vi "KM_Lockin.vi"() -> ()   [LabVIEW 2015]
uses:
  Dropbox/MaxPlanck/HF2LI_KM/MQM Data Transfer_KM.vi
  <vilib>/Utility/file.llb/Write To Spreadsheet File (string).vi
  <vilib>/Utility/file.llb/Write To Spreadsheet File (DBL).vi
  Dropbox/MaxPlanck/HF2LI_KM/String Array Select.vi
  Dropbox/MaxPlanck/HF2LI_KM/Numeric Array Select.vi
panel:
  in  "Tab Control":enum32{"Display Data", "Sweep Arming"}(tab)
  in  "Control":bool=TRUE
  in  "Stop":bool=TRUE
  out "XY Graph":cluster{dbl[], dbl[]}[](graph)
  in  "Display Elements":cluster{"X":bool, "Y":bool, "Name":u16}[](array[cluster]) {"Name" items=["Time (ms)", "Field (T)", "Temperature (K)", "", "HFLI_1.0 Freq (Hz)", "HFLI_1.0 R (V)", "HFLI_1.0 Theta (deg)", "HFLI_1.0 X (mV)", "HFLI_1.0 Y (mV)"]}
  in  "X-Axis":u16(ring) items=["Linear", "Reciprocal", "Log10"]
  in  "Filename":path=path "C:/Users/putkonen.CPFS/Dropbox.lvm"
  in  "Delay (ms)":dbl=2000.0
  out "Data Rate (ms)":u32
  in  "Finish":bool
  in  "Y-Axis":u16(ring) items=["Linear", "Reciprocal", "Log10"]
  in  "Data Recording":bool=TRUE
  in  "DAQ time (ms)":u32=500
  out "Circles":cluster{dbl[], dbl[]}(graph)
  in  "X":u16(ring) items=["Linear", "Reciprocal", "Log10"]
  in  "Y":u16(ring) items=["Linear", "Reciprocal", "Log10"]
  out "Phase":cluster{dbl[], dbl[]}(graph)
  in  "Frequency":u16(ring) items=["Linear", "Reciprocal", "Log10"]
  in  "Theta":u16(ring) items=["Linear", "Reciprocal", "Log10"]
  out "# pts in freq sweep":i32
  out "Data Rate  (ms)":u32
  in  "DAQ time (ms)":u32=50
  in  "Fequency sweep datafile":path=path "C:/Users/putkonen.CPFS/Dropbox.lvm" caption="Filename"
  in  "Start (Hz)":dbl=48.29
  in  "Stop (Hz)":dbl=48.57
  in  "# pts in scan":dbl=100.0
  in  "Bandwidth (Hz)":dbl=10.0
  out "Global Stop":bool
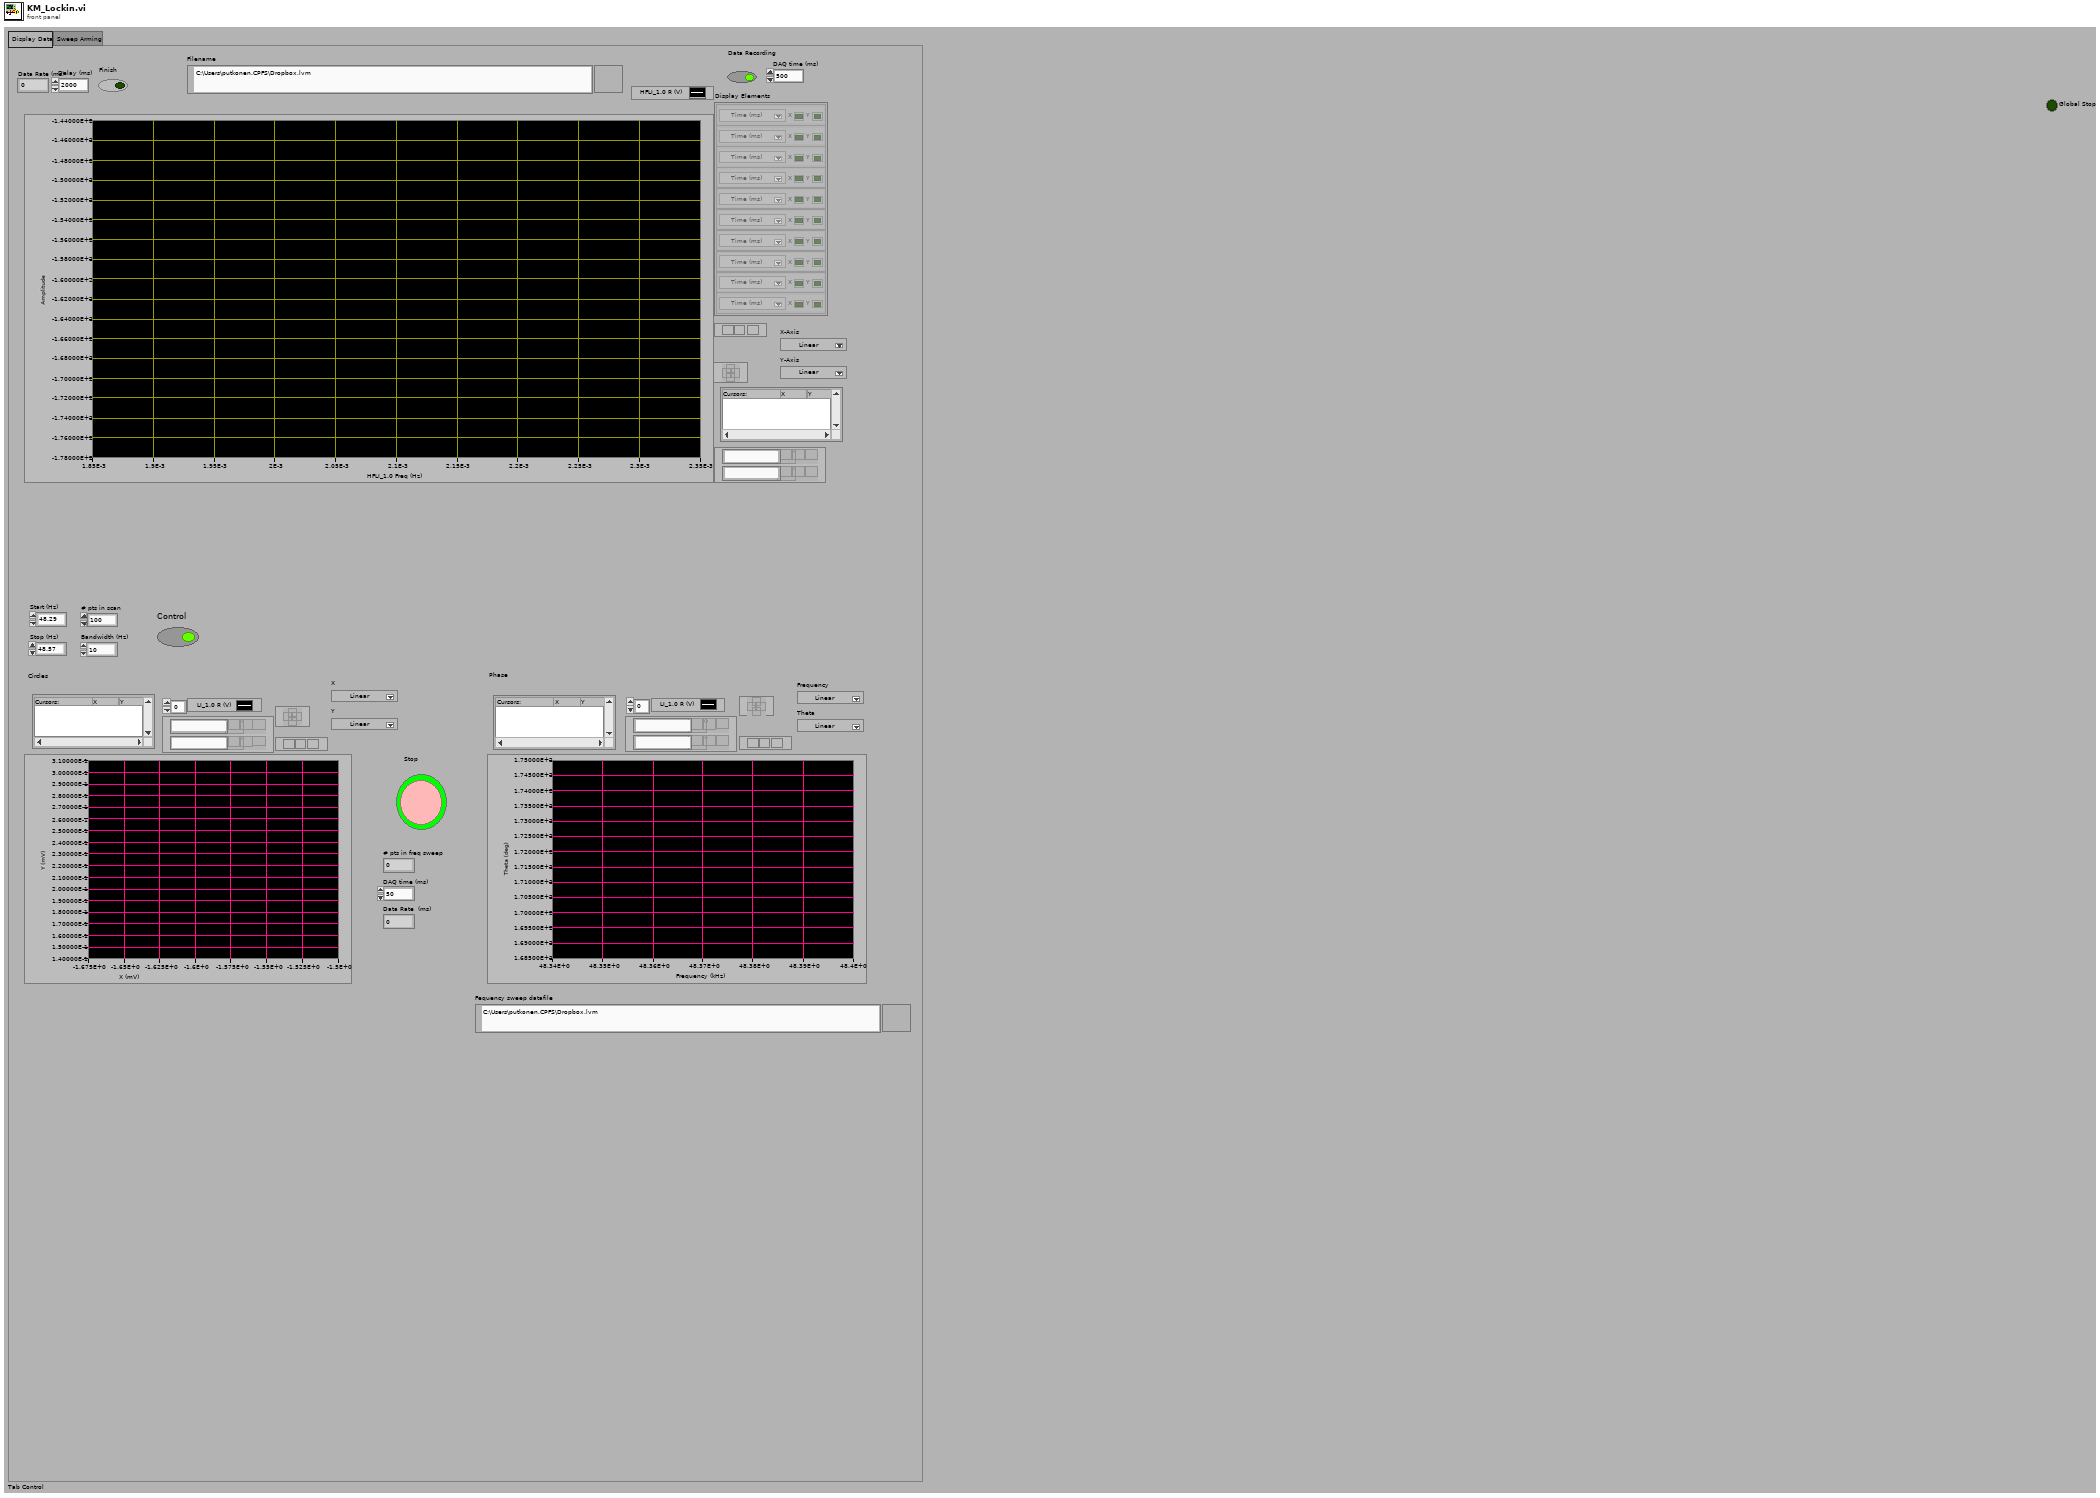
[diagram p1: front panel]
types:
  T1 = typedef "ZI_Frontpanel.ctl" = cluster{"Lockin 1 Demod 0":cluster{"R(V)":dbl, "Theta (deg)":dbl, "Timestamp (ms)":u32}, "Lockin 2 Demod 0":cluster{"R(V)":dbl, "Theta (deg)":dbl, "Timestamp (ms)":u32}, "Lockin 3 Demod 0":cluster{"R(V)":dbl, "Theta (deg)":dbl, "Timestamp (ms)":u32}, "Lockin 4 Demod 0":cluster{"R(V)":dbl, "Theta (deg)":dbl, "Timestamp (ms)":u32}, "Lockin 1 Demod 1":cluster{"R(V)":dbl, "Theta (deg)":dbl, "Timestamp (ms)":u32}, "Lockin 2 Demod 1":cluster{"R(V)":dbl, "Theta (deg)":dbl, "Timestamp (ms)":u32}, "Lockin 3 Demod 1":cluster{"R(V)":dbl, "Theta (deg)":dbl, "Timestamp (ms)":u32}, "Lockin 4 Demod 1":cluster{"R(V)":dbl, "Theta (deg)":dbl, "Timestamp (ms)":u32}, "Lockin 1 Demod 2":cluster{"R(V)":dbl, "Theta (deg)":dbl, "Timestamp (ms)":u32}, "Lockin 1 Demod 3":cluster{"R(V)":dbl, "Theta (deg)":dbl, "Timestamp (ms)":u32}, "LI1 active":bool, "LI2 active":bool, "LI3 active":bool, "LI4 active":bool}
  T2 = typedef "HF_FrontPanel.ctl" = cluster{"Lockin 1 Demod 0":cluster{"R(V)":dbl, "Theta (deg)":dbl, "Frequency (Hz)":dbl, "X (mV)":dbl, "Y (mV)":dbl}, "LI1 active":bool, "Timestamp (ms)":u32}
  T3 = typedef "PPMS_Status.ctl" = cluster{"Field":cluster{"Field (T)":dbl, "Field stable":bool, "Timestamp (ms)":u32}, "Temperature":cluster{"Temperature (K)":dbl, "Temperature stable":bool, "Timestamp (ms)":u32}}
  T4 = cluster{"Request new file":bool, "Sweep variable":u16, "Pause DAQ":bool}
  T5 = typedef "Rotator_Status.ctl" = cluster{"Angle (deg)":dbl, "Stopped":bool, "Timestamp (ms)":u32}
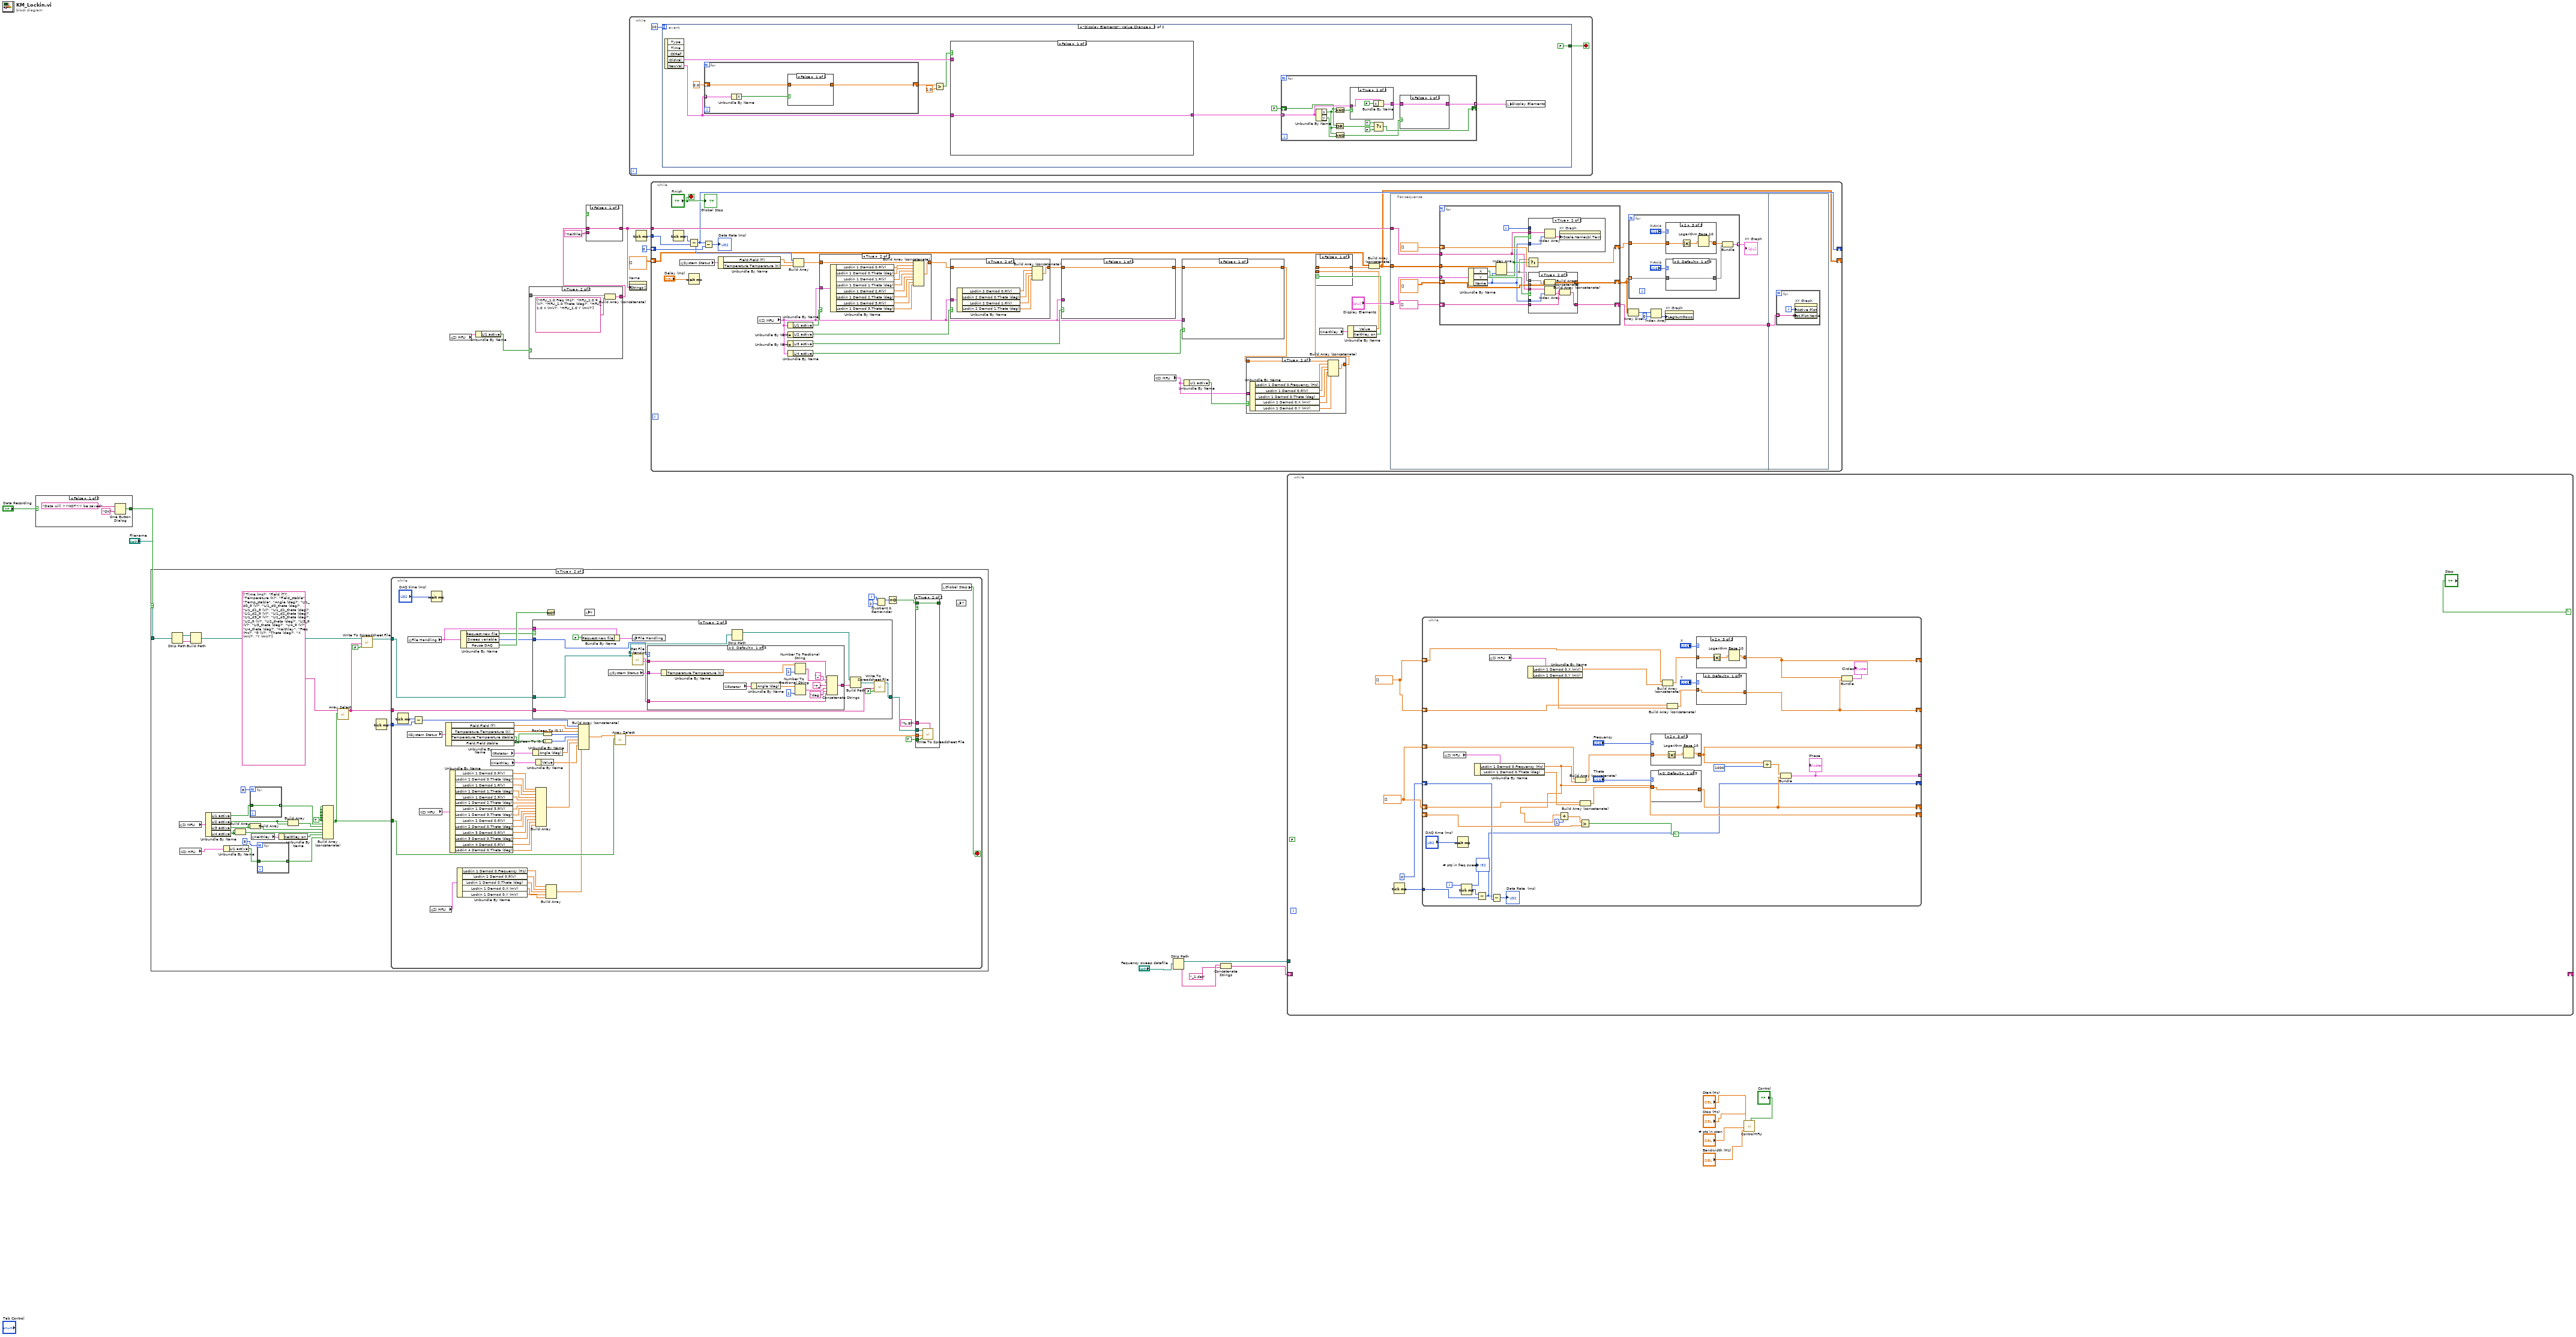
[diagram p0: block diagram]
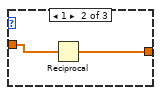
[diagram p2: hidden frame]
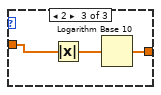
[diagram p3: hidden frame]
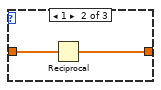
[diagram p5: hidden frame]
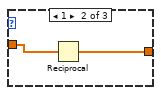
[diagram p6: hidden frame]
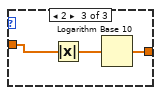
[diagram p7: hidden frame]
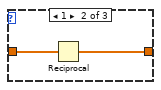
[diagram p9: hidden frame]
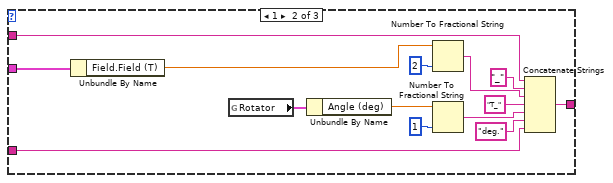
[diagram p13: hidden frame]
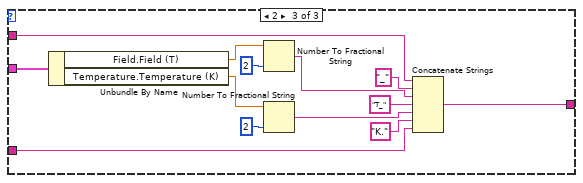
[diagram p14: hidden frame]
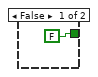
[diagram p15: hidden frame]
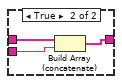
[diagram p17: hidden frame]
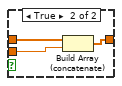
[diagram p19: hidden frame]
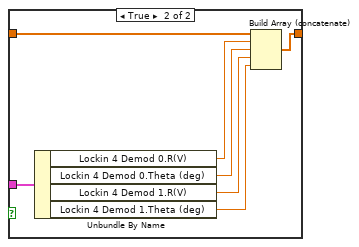
[diagram p20: hidden frame]
diagram:
  n1 = case shown="False" "Data Recording" {
    selector: "Data Recording" -> [_ w26]
    tunnel: [w23 w26] -> w15
    frame False {
      n2 = One Button Dialog(message="Data will >>NOT<< be saved", button name ("OK")="OK") -> (true=w23:bool)
    }
    frame True {
    }
  }
  n3 = case shown="True" w15 {
    tunnel: "Filename" -> [_ w53]
    frame False {
    }
    frame True {
      w45 = TRUE
      n4 = Strip Path(path=w53) -> (stripped path=w49:path, name=w47:string)
      n5 = global read "MQM Data Transfer_KM.vi" "ZI MFLI"() -> (w44:T1)
      n6 = global read "MQM Data Transfer_KM.vi" "ZI HFLI"() -> (w30:T2)
      n7 = Build Path(base path=w49, name or relative path=w47) -> (appended path=w50:path)
      n8 = Unbundle By Name(w44) -> ("LI1 active"=w43:bool, "LI2 active"=w40:bool, "LI3 active"=w39:bool, "LI4 active"=w38:bool)
      n9 = Unbundle By Name(w30) -> ("LI1 active"=w29:bool)
      n10 = Build Array(w38, w38) -> (w35:bool[])
      n11 = for {
        N: 8 -> [_]
        tunnel: w43 -> [w55]
        tunnel: [w55] -> w41 mode=indexing
      }
      n12 = Build Array(w39, w39) -> (w36:bool[])
      n13 = global read "MQM Data Transfer_KM.vi" "Keithley"() -> (w34:cluster{"Value":dbl, "Keithley on":bool})
      n14 = for {
        N: 5 -> [_]
        tunnel: w29 -> [w54]
        tunnel: [w54] -> w27 mode=indexing
      }
      n15 = Unbundle By Name(w34) -> ("Keithley on"=w33:bool)
      n16 = Build Array(w40, w40) -> (w37:bool[])
      n17 = Build Array (concatenate)(w45, w45, w45, w45, w45, w45, w41, w37, w36, w35, w33, w27) -> (w32:bool[])
      n18 = call-poly "Array Select.vi"("Selector array"=w32, "Full array"=string[] ["Time (ms)", "Field (T)", "Temperature (K)", "Field_stable", "Temp_stable", "Angle (deg)", "LI1_d0_R (V)", "LI1_d0_theta (deg)", "LI1_d1_R (V)", "LI1_d1_theta (deg)", "LI1_d2_R (V)", "LI1_d2_theta (deg)", "LI1_d3_R (V)", "LI1_d3_theta (deg)", "LI2_R (V)", "LI2_theta (deg)", "LI3_R (V)", "LI3_theta (deg)", "LI4_R (V)", "LI4_theta (deg)", "Keithley", "Freq (Hz)", "R (V)", "Theta (deg)", "X (mV)", "Y (mV)"]) -> ("Array"=w31:string[])  [unwired: 9 in]
      n19 = call-poly <vilib>:"Write To Spreadsheet File.vi"("append to file? (new file:F)"=FALSE, "1D data"=w31, "file path (dialog if empty)"=w50) -> ("new file path (Not A Path if cancelled)"=w48:path)  [unwired: 5 in]
      n20 = Tick Count (ms)() -> (millisecond timer value=w52:u32)
      n21 = while {
        tunnel: w52 -> [w110]
        tunnel: w48 -> [w70]
        tunnel: w32 -> [w77]
        tunnel: w31 -> [w67]
        i -> [w76]
        stop <- w102 stop-if-true
        n22 = Tick Count (ms)() -> (millisecond timer value=w108:u32)
        n23 = global read "MQM Data Transfer_KM.vi" "System Status"() -> (w109:T3)
        n24 = global read "MQM Data Transfer_KM.vi" "File Handling"() -> (w66:T4)
        n25 = Subtract(x=w108, y=w110) -> (x-y=w107:u32)
        n26 = global read "MQM Data Transfer_KM.vi" "ZI MFLI"() -> (w98:T1)
        n27 = global read "MQM Data Transfer_KM.vi" "ZI HFLI"() -> (w63:T2)
        n28 = Wait (ms)(milliseconds to wait="DAQ time (ms)") -> ()  [unwired: 1 out]
        n29 = Unbundle By Name(w109) -> ("Field.Field (T)"=w106:dbl, "Temperature.Temperature (K)"=w105:dbl, "Temperature.Temperature stable"=w86:bool, "Field.Field stable"=w88:bool)
        n30 = Unbundle By Name(w98) -> ("Lockin 1 Demod 0.R(V)"=w97:dbl, "Lockin 1 Demod 0.Theta (deg)"=w96:dbl, "Lockin 1 Demod 1.R(V)"=w95:dbl, "Lockin 1 Demod 1.Theta (deg)"=w94:dbl, "Lockin 1 Demod 2.R(V)"=w93:dbl, "Lockin 1 Demod 2.Theta (deg)"=w92:dbl, "Lockin 1 Demod 3.R(V)"=w91:dbl, "Lockin 1 Demod 3.Theta (deg)"=w90:dbl, "Lockin 2 Demod 0.R(V)"=w89:dbl, "Lockin 2 Demod 0.Theta (deg)"=w82:dbl, "Lockin 3 Demod 0.R(V)"=w81:dbl, "Lockin 3 Demod 0.Theta (deg)"=w80:dbl, "Lockin 4 Demod 0.R(V)"=w79:dbl, "Lockin 4 Demod 0.Theta (deg)"=w78:dbl)
        n31 = Unbundle By Name(w63) -> ("Lockin 1 Demod 0.Frequency (Hz)"=w62:dbl, "Lockin 1 Demod 0.R(V)"=w61:dbl, "Lockin 1 Demod 0.Theta (deg)"=w60:dbl, "Lockin 1 Demod 0.X (mV)"=w59:dbl, "Lockin 1 Demod 0.Y (mV)"=w58:dbl)
        n32 = Unbundle By Name(w66) -> ("Request new file"=w71:bool, "Sweep variable"=w68:u16, "Pause DAQ"=w73:bool)
        n33 = global read "MQM Data Transfer_KM.vi" "Keithley"() -> (w99:cluster{"Value":dbl, "Keithley on":bool})
        n34 = global read "MQM Data Transfer_KM.vi" "Rotator"() -> (w100:T5)
        n35 = case shown="True" w71 {
          tunnel: w70 -> [w111 w122]
          tunnel: [w111 w115] -> w69
          tunnel: w68 -> [_ w124]
          tunnel: w67 -> [_ w117]
          tunnel: w66 -> [_ w114]
          frame False {
          }
          frame True {
            n36 = Bundle By Name(cluster=w114, "Request new file"=FALSE) -> (w112:T4)
            n37 = global read "MQM Data Transfer_KM.vi" "System Status"() -> (w123:T3)
            n38 = global write "MQM Data Transfer_KM.vi" "File Handling"(w112) -> ()
            n39 = call <vilib>:"Get File Extension.vi"("file"=w122) -> ("filename without extension"=w121:string, "lowercase file extension"=w120:string)  [unwired: 6 in, 3 out]
            n40 = case shown="0, Default" w124 {
              tunnel: w123 -> [w139 w148 w159]
              tunnel: w121 -> [w136 w149 w161]
              tunnel: w120 -> [w126 w140 w154]
              tunnel: [w132 w146 w160] -> w119
              frame 0, Default {
                n41 = Unbundle By Name(w139) -> ("Temperature.Temperature (K)"=w138:dbl)
                n42 = global read "MQM Data Transfer_KM.vi" "Rotator"() -> (w131:T5)
                n43 = Unbundle By Name(w131) -> ("Angle (deg)"=w129:dbl)
                n44 = Number To Fractional String(number=w138, precision (6)=i16 2) -> (F-format string=w134:string)  [unwired: 2 in]
                n45 = Number To Fractional String(number=w129, precision (6)=i16 1) -> (F-format string=w128:string)  [unwired: 2 in]
                n46 = Concatenate Strings(w136, "_", w134, "T_", w128, "deg." ("string"), w126) -> (w132:string)
              }
              frame 1 {
                n47 = Unbundle By Name(w148) -> ("Field.Field (T)"=w147:dbl)
                n48 = global read "MQM Data Transfer_KM.vi" "Rotator"() -> (w145:T5)
                n49 = Unbundle By Name(w145) -> ("Angle (deg)"=w143:dbl)
                n50 = Number To Fractional String(number=w147, precision (6)=i16 2) -> (F-format string=w151:string)  [unwired: 2 in]
                n51 = Number To Fractional String(number=w143, precision (6)=i16 1) -> (F-format string=w142:string)  [unwired: 2 in]
                n52 = Concatenate Strings(w149, "_", w151, "T_", w142, "deg." ("string"), w140) -> (w146:string)
              }
              frame 2 {
                n53 = Unbundle By Name(w159) -> ("Field.Field (T)"=w166:dbl, "Temperature.Temperature (K)"=w157:dbl)
                n54 = Number To Fractional String(number=w166, precision (6)=i16 2) -> (F-format string=w163:string)  [unwired: 2 in]
                n55 = Number To Fractional String(number=w157, precision (6)=i16 2) -> (F-format string=w156:string)  [unwired: 2 in]
                n56 = Concatenate Strings(w161, "_", w163, "T_", w156, "K." ("string"), w154) -> (w160:string)
              }
            }
            n57 = Strip Path(path=w122) -> (stripped path=w125:path)  [unwired: 1 out]
            n58 = Build Path(base path=w125, name or relative path=w119) -> (appended path=w116:path)
            n59 = call-poly <vilib>:"Write To Spreadsheet File.vi"("append to file? (new file:F)"=FALSE, "1D data"=w117, "file path (dialog if empty)"=w116) -> ("new file path (Not A Path if cancelled)"=w115:path)  [unwired: 5 in]
          }
        }
        n60 = Unbundle By Name(w100) -> ("Angle (deg)"=w84:dbl)
        n61 = Build Array(w97, w96, w95, w94, w93, w92, w91, w90, w89, w82, w81, w80, w79, w78) -> (w83:dbl[])
        n62 = Unbundle By Name(w99) -> ("Value"=w64:dbl)
        n63 = Boolean To (0,1)(Boolean=w88) -> (0, 1=w87:i16)
        n64 = Boolean To (0,1)(Boolean=w86) -> (0, 1=w85:i16)
        n65 = Not(x=w73) -> ()  [unwired: 1 out]
        n66 = Build Array(w62, w61, w60, w59, w58) -> (w57:dbl[])
        n67 = Build Array (concatenate)(w107, w106, w105, w87, w85, w84, w83, w64, w57) -> (w65:dbl[])
        n68 = local read item#-1() -> ()  [unwired: 1 in]
        n69 = call-poly "Array Select.vi"("Selector array"=w77, "Full array"=w65) -> ("Array"=w56:dbl[])  [unwired: 9 in]
        n70 = Quotient & Remainder(x=w76, y=2) -> (x-y*floor(x/y)=w74:i32)  [unwired: 1 out]
        n71 = Equal To 0?(x=w74) -> (x = 0?=w72:bool)
        n72 = case shown="True" {
          selector: _ -> [_ _]
          tunnel: TRUE ("append to file? (new file:F)") -> [_ w172]
          tunnel: "%.8f" ("format (%.3f)") -> [_ w171]
          tunnel: w56 -> [_ w170]
          tunnel: w72 -> [_ w169]
          tunnel: [FALSE w169] -> _
          tunnel: w69 -> [_ w168]
          frame False {
          }
          frame True {
            n73 = call-poly <vilib>:"Write To Spreadsheet File.vi"("format (%.3f)"=w171, "append to file? (new file:F)"=w172, "1D data"=w170, "file path (dialog if empty)"=w168) -> ()  [unwired: 4 in, 1 out]
          }
        }
        n74 = local read "Global Stop"() -> (w102:bool)
        n75 = local read item#-1() -> ()  [unwired: 1 in]
      }
    }
  }
  n76 = global read "MQM Data Transfer_KM.vi" "ZI HFLI"() -> (w13:T2)
  n77 = Unbundle By Name(w13) -> ("LI1 active"=w12:bool)
  n78 = case shown="True" w12 {
    tunnel: _ -> [w173 w176]
    tunnel: [w173 w174] -> w11
    frame False {
    }
    frame True {
      n79 = Build Array (concatenate)(w176, string[] ["HFLI_1.0 Freq (Hz)", "HFLI_1.0 R (V)", "HFLI_1.0 Theta (deg)", "HFLI_1.0 X (mV)", "HFLI_1.0 Y (mV)"]) -> (w174:string[])
    }
  }
  n80 = case shown="False" w17 {
    tunnel: w11 -> [w177 w180]
    tunnel: "Keithley" -> [_ w179]
    tunnel: [w177 w178] -> w18
    frame False {
    }
    frame True {
      n81 = Build Array (concatenate)(w180, w179) -> (w178:string[])
    }
  }
  n82 = while {
    stop <- w181 stop-if-true
    n83 = event shown="[1] \"Display Elements\": Value Change" {
      selector: _ -> [_ _]
      dyn-events: _ -> [_ _]
      timeout: 20 -> [_ _]
      tunnel: [w183 FALSE] -> w181
      event Timeout {
        n84 = event-data() -> ()  [unwired: 1 in, 2 out]
        n85 = local read "Global Stop"() -> (w184:bool)
        n86 = case shown="False" w184 {
          tunnel: [FALSE TRUE] -> w183
          frame False {
          }
          frame True {
          }
        }
      }
      event "Display Elements": Value Change {
        n87 = event-data() -> ("OldVal"=w194:cluster{"X":bool, "Y":bool, "Name":u16}[], "NewVal"=w192:cluster{"X":bool, "Y":bool, "Name":u16}[])  [unwired: 1 in, 3 out]
        n88 = for {
          tunnel: w192 -> [w217] mode=indexing
          shift-right: [w215] -> w190
          shift-left: 0.0 -> [w214]
          n89 = Unbundle By Name(w217) -> ("X"=w216:bool)
          n90 = case shown="False" w216 {
            tunnel: [w218 w220] -> w215
            tunnel: w214 -> [w218 w219]
            frame False {
            }
            frame True {
              n91 = Increment(x=w219) -> (x+1=w220:dbl)
            }
          }
        }
        n92 = Greater?(x=w190, y=1.0) -> (0:w188:bool)
        n93 = case shown="False" w188 {
          tunnel: w194 -> [_ w200]
          tunnel: [w197 w199] -> w193
          tunnel: w192 -> [w197 w198]
          frame False {
          }
          frame True {
            n94 = for {
              tunnel: w198 -> [w203] mode=indexing
              tunnel: w200 -> [w207] mode=indexing
              tunnel: [w202] -> w199 mode=indexing
              n95 = Unbundle By Name(w207) -> ("X"=w206:bool)
              n96 = Unbundle By Name(w203) -> ("X"=w205:bool)
              n97 = Not(x=w206) -> (.not. x?=w204:bool)
              n98 = And(x=w204, y=w205) -> (x .and. y?=w201:bool)
              n99 = case shown="True" w201 {
                tunnel: [w208 w212] -> w202
                tunnel: w203 -> [w210 w211]
                frame False {
                  n100 = Bundle By Name(cluster=w210, "X"=FALSE) -> (w208:cluster{"X":bool, "Y":bool, "Name":u16})
                }
                frame True {
                  n101 = Bundle By Name(cluster=w211, "X"=TRUE) -> (w212:cluster{"X":bool, "Y":bool, "Name":u16})
                }
              }
            }
          }
        }
        n102 = for {
          tunnel: w193 -> [w231] mode=indexing
          shift-right: [w227] -> _
          shift-left: FALSE ("X") -> [w230]
          tunnel: [w221] -> w195 mode=indexing
          n103 = Unbundle By Name(w231) -> ("X"=w225:bool, "Y"=w224:bool)
          n104 = Or(x=w230, y=w225) -> (x .or. y?=w229:bool)
          n105 = And(x=w230, y=w225) -> (x .and. y?=w232:bool)
          n106 = And(x=w225, y=w224) -> (x .and. y?=w223:bool)
          n107 = case shown="True" w232 {
            tunnel: w231 -> [w237 w240]
            tunnel: [w237 w238] -> w222
            frame False {
            }
            frame True {
              n108 = Bundle By Name(cluster=w240, "X"=FALSE) -> (w238:cluster{"X":bool, "Y":bool, "Name":u16})
            }
          }
          n109 = Select(t=TRUE, s=w229, f=FALSE) -> (s? t:f=w227:bool)
          n110 = case shown="False" w223 {
            tunnel: w222 -> [w233 w236]
            tunnel: [w233 w235] -> w221
            frame False {
            }
            frame True {
              n111 = Bundle By Name(cluster=w236, "Y"=FALSE) -> (w235:cluster{"X":bool, "Y":bool, "Name":u16})
            }
          }
        }
        n112 = local write "Display Elements"(w195) -> ()
      }
    }
  }
  n113 = property on="Name" class="Ring (strict)"("Strings []"=w18) -> ()  [unwired: 2 in, 2 out]
  n114 = Tick Count (ms)() -> (millisecond timer value=w22:u32)
  n115 = while {
    tunnel: w22 -> [w271]
    shift-right: [w262] -> _
    shift-left: 0 -> [w270]
    tunnel: w18 -> [w264]
    shift-right: [w249] -> _
    shift-left: dbl[][] [] -> [w250]
    stop <- "Finish" stop-if-true
    n116 = Tick Count (ms)() -> (millisecond timer value=w272:u32)
    n117 = global read "MQM Data Transfer_KM.vi" "System Status"() -> (w253:T3)
    n118 = Subtract(x=w272, y=w271) -> (x-y=w262:u32)
    n119 = Wait (ms)(milliseconds to wait="Delay (ms)") -> ()  [unwired: 1 out]
    n120 = Subtract(x=w262, y=w270) -> (x-y=→"Data Rate (ms)":u32)
    n121 = Unbundle By Name(w253) -> ("Field.Field (T)"=w252:dbl, "Temperature.Temperature (K)"=w251:dbl)
    n122 = global read "MQM Data Transfer_KM.vi" "ZI MFLI"() -> (w255:T1)
    n123 = Unbundle By Name(w255) -> ("LI1 active"=w263:bool)
    n124 = Unbundle By Name(w255) -> ("LI2 active"=w260:bool)
    n125 = Unbundle By Name(w255) -> ("LI3 active"=w258:bool)
    n126 = Unbundle By Name(w255) -> ("LI4 active"=w256:bool)
    n127 = Build Array(w262, w252, w251) -> (w261:dbl[])
    n128 = case shown="True" w263 {
      tunnel: w255 -> [_ w321]
      tunnel: w261 -> [w310 w320]
      tunnel: [w310 w311] -> w259
      frame False {
      }
      frame True {
        n129 = Unbundle By Name(w321) -> ("Lockin 1 Demod 0.R(V)"=w319:dbl, "Lockin 1 Demod 0.Theta (deg)"=w318:dbl, "Lockin 1 Demod 1.R(V)"=w317:dbl, "Lockin 1 Demod 1.Theta (deg)"=w316:dbl, "Lockin 1 Demod 2.R(V)"=w315:dbl, "Lockin 1 Demod 2.Theta (deg)"=w314:dbl, "Lockin 1 Demod 3.R(V)"=w313:dbl, "Lockin 1 Demod 3.Theta (deg)"=w312:dbl)
        n130 = Build Array (concatenate)(w320, w319, w318, w317, w316, w315, w314, w313, w312) -> (w311:dbl[])
      }
    }
    n131 = case shown="True" w260 {
      tunnel: w255 -> [_ w309]
      tunnel: w259 -> [w302 w304]
      tunnel: [w302 w303] -> w257
      frame False {
      }
      frame True {
        n132 = Unbundle By Name(w309) -> ("Lockin 2 Demod 0.R(V)"=w308:dbl, "Lockin 2 Demod 0.Theta (deg)"=w307:dbl, "Lockin 2 Demod 1.R(V)"=w306:dbl, "Lockin 2 Demod 1.Theta (deg)"=w305:dbl)
        n133 = Build Array (concatenate)(w304, w308, w307, w306, w305) -> (w303:dbl[])
      }
    }
    n134 = case shown="False" w258 {
      tunnel: w255 -> [_ w301]
      tunnel: w257 -> [w294 w296]
      tunnel: [w294 w295] -> w254
      frame False {
      }
      frame True {
        n135 = Unbundle By Name(w301) -> ("Lockin 3 Demod 0.R(V)"=w300:dbl, "Lockin 3 Demod 0.Theta (deg)"=w299:dbl, "Lockin 3 Demod 1.R(V)"=w298:dbl, "Lockin 3 Demod 1.Theta (deg)"=w297:dbl)
        n136 = Build Array (concatenate)(w296, w300, w299, w298, w297) -> (w295:dbl[])
      }
    }
    n137 = global read "MQM Data Transfer_KM.vi" "ZI HFLI"() -> (w243:T2)
    n138 = case shown="False" w256 {
      tunnel: w255 -> [_ w293]
      tunnel: w254 -> [w286 w288]
      tunnel: [w286 w287] -> w241
      frame False {
      }
      frame True {
        n139 = Unbundle By Name(w293) -> ("Lockin 4 Demod 0.R(V)"=w292:dbl, "Lockin 4 Demod 0.Theta (deg)"=w291:dbl, "Lockin 4 Demod 1.R(V)"=w290:dbl, "Lockin 4 Demod 1.Theta (deg)"=w289:dbl)
        n140 = Build Array (concatenate)(w288, w292, w291, w290, w289) -> (w287:dbl[])
      }
    }
    n141 = Unbundle By Name(w243) -> ("LI1 active"=w244:bool)
    n142 = case shown="True" w244 {
      tunnel: w243 -> [_ w281]
      tunnel: w241 -> [w273 w274]
      tunnel: [w273 w276] -> w242
      frame False {
      }
      frame True {
        n143 = Unbundle By Name(w281) -> ("Lockin 1 Demod 0.Frequency (Hz)"=w280:dbl, "Lockin 1 Demod 0.R(V)"=w279:dbl, "Lockin 1 Demod 0.Theta (deg)"=w278:dbl, "Lockin 1 Demod 0.X (mV)"=w277:dbl, "Lockin 1 Demod 0.Y (mV)"=w275:dbl)
        n144 = Build Array (concatenate)(w274, w280, w279, w278, w277, w275) -> (w276:dbl[])
      }
    }
    n145 = global read "MQM Data Transfer_KM.vi" "Keithley"() -> (w248:cluster{"Value":dbl, "Keithley on":bool})
    n146 = Unbundle By Name(w248) -> ("Value"=w247:dbl, "Keithley on"=w245:bool)
    n147 = case shown="False" w245 {
      tunnel: w242 -> [w282 w285]
      tunnel: w247 -> [_ w284]
      tunnel: [w282 w283] -> w246
      frame False {
      }
      frame True {
        n148 = Build Array (concatenate)(w285, w284) -> (w283:dbl[])
      }
    }
    n149 = Build Array (concatenate)(w250, w246) -> (w249:dbl[][])
    n150 = flat-sequence {
      tunnel: "Display Elements" -> [w324]
      tunnel: [w328] -> w268
      tunnel: w264 -> [w322]
      tunnel: w249 -> [w323]
      tunnel: w268 -> [w381]
      frame #0 {
        n151 = for {
          tunnel: w324 -> [w361] mode=indexing
          shift-right: [w367] -> w334
          shift-left: dbl[] [] -> [w366]
          shift-right: [w355] -> w332
          shift-left: dbl[][] [] -> [w363]
          shift-right: [w359] -> w328
          shift-left: string[] [] -> [w358]
          tunnel: w322 -> [w354]
          tunnel: w323 -> [w356]
          i -> [w357]
          n152 = Unbundle By Name(w361) -> ("X"=w362:bool, "Y"=w365:bool, "Name"=w360:u16)
          n153 = Index Array(array=w356, index (col)=w360) -> (element=w364:dbl[])  [unwired: 1 in]
          n154 = Select(t=w364, s=w362, f=w366) -> (s? t:f=w367:dbl[])
          n155 = case shown="True" w362 {
            tunnel: w360 -> [_ w370]
            tunnel: w357 -> [_ _]
            tunnel: w354 -> [_ w368]
            frame False {
            }
            frame True {
              n156 = Index Array(array=w368, index=w370) -> (element=w369:string)
              n157 = property on="XY Graph" class="XYGraph (strict)"("XScale.NameLbl.Text"=w369) -> ()  [unwired: 2 in, 2 out]
            }
          }
          n158 = case shown="True" w365 {
            tunnel: w364 -> [_ w373]
            tunnel: w363 -> [w371 w380]
            tunnel: [w371 w379] -> w355
            tunnel: w360 -> [_ w378]
            tunnel: [w372 w376] -> w359
            tunnel: w358 -> [w372 w375]
            tunnel: w354 -> [_ w374]
            frame False {
            }
            frame True {
              n159 = Build Array (concatenate)(w380, w373) -> (w379:dbl[][])
              n160 = Index Array(array=w374, index=w378) -> (element=w377:string)
              n161 = Build Array (concatenate)(w375, w377) -> (w376:string[])
            }
          }
        }
        n162 = Array Size(array=w332) -> (size(s)=w331:i32[])
        n163 = for {
          tunnel: w332 -> [w338] mode=indexing
          tunnel: w334 -> [w340]
          tunnel: [w341] -> w333 mode=indexing
          n164 = case shown="2" "X-Axis" {
            tunnel: w340 -> [w348 w350 w353]
            tunnel: [w348 w349 w352] -> w339
            frame 0, Default {
            }
            frame 1 {
              n165 = Reciprocal(x=w350) -> (1/x=w349:dbl[])
            }
            frame 2 {
              n166 = Absolute Value(x=w353) -> (abs(x)=w351:dbl[])
              n167 = Logarithm Base 10(1:w351) -> (0:w352:dbl[])
            }
          }
          n168 = case shown="0, Default" "Y-Axis" {
            tunnel: w338 -> [w342 w344 w347]
            tunnel: [w342 w343 w346] -> w335
            frame 0, Default {
            }
            frame 1 {
              n169 = Reciprocal(x=w344) -> (1/x=w343:dbl[])
            }
            frame 2 {
              n170 = Absolute Value(x=w347) -> (abs(x)=w345:dbl[])
              n171 = Logarithm Base 10(1:w345) -> (0:w346:dbl[])
            }
          }
          n172 = Bundle(w339, w335) -> (w341:cluster{dbl[], dbl[]})  [unwired: 1 in]
        }
        "XY Graph" <- w333
        n173 = Index Array(array=w331, index=0) -> (element=w329:i32)
        n174 = property on="XY Graph" class="XYGraph (strict)"("LegNumRows"=w329) -> ()  [unwired: 2 in, 2 out]
      }
      frame #1 {
        n175 = for {
          tunnel: w381 -> [w382] mode=indexing
          i -> [w383]
          n176 = property on="XY Graph" class="XYGraph (strict)"("Active Plot"=w383, "Plot.Plot Name"=w382) -> ()  [unwired: 2 in, 2 out]
        }
      }
    }
    "Global Stop" <- "Finish"
  }
  n177 = Strip Path(path="Fequency sweep datafile") -> (stripped path=w6:path, name=w10:string)
  n178 = Concatenate Strings(w10, "_1.dat") -> (w7:string)
  n179 = while {
    shift-right: _ -> [_]
    shift-left: w7 -> [_]
    tunnel: w6 -> [_]
    stop <- "Stop" continue-if-true
    (unwired) FALSE ("Save current freq scan")
    w384 = dbl[] []
    w387 = dbl[] []
    n180 = Tick Count (ms)() -> (millisecond timer value=w386:u32)
    n181 = while {
      shift-right: [w393] -> _
      shift-left: w387 -> [w391]
      shift-right: [w394] -> _
      shift-left: w387 -> [w390]
      shift-right: [w415] -> _
      shift-left: _ -> [w416]
      tunnel: [w418] -> _
      tunnel: w386 -> [w410]
      shift-right: [w389] -> _
      shift-left: 0 -> [w408]
      shift-right: [w398] -> _
      shift-left: w384 -> [w397]
      shift-right: [w396] -> _
      shift-left: w384 -> [w399]
      i -> [w395]
      stop <- w392 continue-if-true
      n182 = global read "MQM Data Transfer_KM.vi" "ZI HFLI"() -> (w421:T2)
      n183 = Wait (ms)(milliseconds to wait="DAQ time (ms)") -> ()  [unwired: 1 out]
      n184 = Tick Count (ms)() -> (millisecond timer value=w412:u32)
      n185 = Unbundle By Name(w421) -> ("Lockin 1 Demod 0.Frequency (Hz)"=w415:dbl, "Lockin 1 Demod 0.Theta (deg)"=w417:dbl)
      n186 = Subtract(x=w412, y=w410) -> (x-y=w389:u32)
      n187 = global read "MQM Data Transfer_KM.vi" "ZI HFLI"() -> (w403:T2)
      n188 = Subtract(x=w389, y=w408) -> (x-y=→"Data Rate  (ms)":u32)
      n189 = Unbundle By Name(w403) -> ("Lockin 1 Demod 0.X (mV)"=w401:dbl, "Lockin 1 Demod 0.Y (mV)"=w400:dbl)
      n190 = Add(x=w415, y=1) -> (x+y=w414:dbl)
      n191 = Build Array (concatenate)(w390, w415) -> (w423:dbl[])
      n192 = Greater?(x=w414, y=w416) -> (0:w392:bool)
      n193 = Build Array (concatenate)(w391, w417) -> (w422:dbl[])
      n194 = case shown="2" "Frequency" {
        tunnel: w423 -> [w444 w446 w449]
        tunnel: [w444 w445 w448] -> w394
        frame 0, Default {
        }
        frame 1 {
          n195 = Reciprocal(x=w446) -> (1/x=w445:dbl[])
        }
        frame 2 {
          n196 = Absolute Value(x=w449) -> (abs(x)=w447:dbl[])
          n197 = Logarithm Base 10(1:w447) -> (0:w448:dbl[])
        }
      }
      n198 = case shown="0, Default" "Theta" {
        tunnel: [w438 w440 w443] -> w393
        tunnel: w422 -> [w438 w439 w441]
        frame 0, Default {
        }
        frame 1 {
          n199 = Reciprocal(x=w439) -> (1/x=w440:dbl[])
        }
        frame 2 {
          n200 = Absolute Value(x=w441) -> (abs(x)=w442:dbl[])
          n201 = Logarithm Base 10(1:w442) -> (0:w443:dbl[])
        }
      }
      n202 = Build Array (concatenate)(w397, w401) -> (w405:dbl[])
      n203 = Build Array (concatenate)(w399, w400) -> (w404:dbl[])
      n204 = case shown="2" "X" {
        tunnel: w405 -> [w432 w434 w437]
        tunnel: [w432 w433 w436] -> w398
        frame 0, Default {
        }
        frame 1 {
          n205 = Reciprocal(x=w434) -> (1/x=w433:dbl[])
        }
        frame 2 {
          n206 = Absolute Value(x=w437) -> (abs(x)=w435:dbl[])
          n207 = Logarithm Base 10(1:w435) -> (0:w436:dbl[])
        }
      }
      n208 = case shown="0, Default" "Y" {
        tunnel: [w426 w428 w431] -> w396
        tunnel: w404 -> [w426 w427 w429]
        frame 0, Default {
        }
        frame 1 {
          n209 = Reciprocal(x=w427) -> (1/x=w428:dbl[])
        }
        frame 2 {
          n210 = Absolute Value(x=w429) -> (abs(x)=w430:dbl[])
          n211 = Logarithm Base 10(1:w430) -> (0:w431:dbl[])
        }
      }
      n212 = Divide(x=w394, y=1000) -> (x/y=w419:dbl[])
      n213 = Bundle(w419, w393) -> (w418:cluster{dbl[], dbl[]})  [unwired: 1 in]
      "Phase" <- w418
      n214 = Bundle(w398, w396) -> (→"Circles":cluster{dbl[], dbl[]})  [unwired: 1 in]
      "# pts in freq sweep" <- w395
    }
  }
  n215 = call "ControlHFLI.vi"("Sweep"="Control", "Bandwidth (Hz)"="Bandwidth (Hz)", "Number of Points"="# pts in scan", "Stop (Hz)"="Stop (Hz)", "Start (Hz)"="Start (Hz)") -> ()  [unwired: 7 in]
